vi "Enumerate Compute Nodes.vi"(8 "error in":errorcluster, 11 "request data":T3) -> (0 "error out":errorcluster, 3 "response data":T1)   [LabVIEW 2021, in "NI Discovery V1 Client.lvlib"]
uses:
  NI Discovery V1 Client.lvlib
  TypeDefs/gRPC Client Cache FGV Action.ctl
  gRPC/Generated APIs/ni/measurementlink/discovery/v1/ni.measurementlink.discovery.v1.api.lvlib
  gRPC/Generated APIs/ni/measurementlink/discovery/v1/RPC Messages/ni_measurementlink_discovery_v1_EnumerateComputeNodesRequest.ctl
  gRPC/Generated APIs/ni/measurementlink/discovery/v1/RPC Messages/ni_measurementlink_discovery_v1_ComputeNodeDescriptor.ctl
  gRPC/Generated APIs/ni/measurementlink/discovery/v1/RPC Messages/ni_measurementlink_discovery_v1_EnumerateComputeNodesResponse.ctl
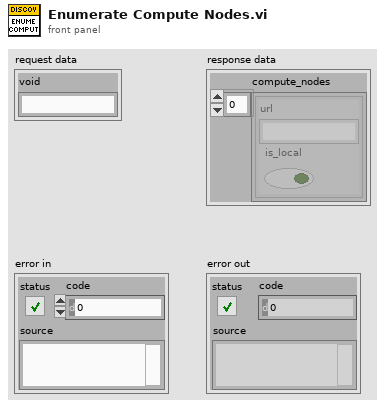
[diagram p1: front panel]
types:
  T1 = typedef "ni.measurementlink.discovery.v1.api.lvlib/ni_measurementlink_discovery_v1_EnumerateComputeNodesResponse.ctl" = cluster{"compute_nodes":T2[]}
  T2 = typedef "ni.measurementlink.discovery.v1.api.lvlib/ni_measurementlink_discovery_v1_ComputeNodeDescriptor.ctl" = cluster{"url":string, "is_local":bool}
  T3 = typedef "ni.measurementlink.discovery.v1.api.lvlib/ni_measurementlink_discovery_v1_EnumerateComputeNodesRequest.ctl" = cluster{"void":string}
  T4 = typedef "NI Discovery V1 Client.lvlib/gRPC Client Cache FGV Action.ctl" = enum16{"Get Client", "Recreate Client", "Destroy Client", "Update ClusterId"}
  T5 = typedef "grpc-lvsupport-release.lvlib/grpcId.ctl" = u64
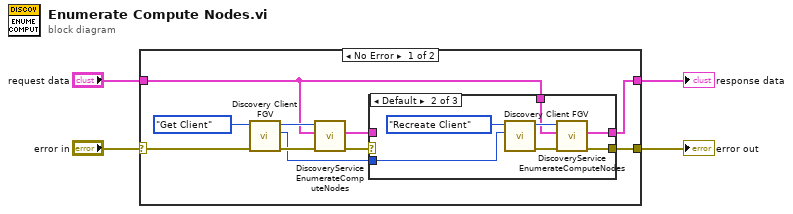
[diagram p0: block diagram]
diagram:
  n1 = case shown="No Error" "error in" {
    selector: "error in" -> [w14 w24]
    tunnel: [w9 w24] -> w3
    tunnel: [w8 _] -> w1
    tunnel: "request data" -> [w5 _]
    frame No Error {
      n2 = call "Discovery Client FGV.vi"("error in"=w14, "action"=gRPC_Client_Cache_FGV_Action."Get Client") -> ("error out"=w12:errorcluster, "unique id out"=w6:u64, "grpc client id"=w11:T5)  [unwired: 6 in, 1 out]
      n3 = call "DiscoveryService EnumerateComputeNodes.vi"("error in"=w12, "Request Data"=w5, "gRPC ID"=w11) -> ("error out"=w10:errorcluster, "Response Data"=w7:T1)  [unwired: 6 in, 1 out]
      n4 = case shown="Default" w10 {
        selector: w10 -> [w16 _ _]
        tunnel: [w16 w20 _] -> w9
        tunnel: [w15 w19 _] -> w8
        tunnel: w7 -> [w15 _ _]
        tunnel: w5 -> [_ w18 _]
        tunnel: w6 -> [_ w17 _]
        frame No Error {
        }
        frame Default {
          n5 = call "Discovery Client FGV.vi"("unique id in"=w17, "action"=gRPC_Client_Cache_FGV_Action."Recreate Client") -> ("error out"=w21:errorcluster, "grpc client id"=w22:T5)  [unwired: 6 in, 2 out]
          n6 = call "DiscoveryService EnumerateComputeNodes.vi"("error in"=w21, "Request Data"=w18, "gRPC ID"=w22) -> ("error out"=w20:errorcluster, "Response Data"=w19:T1)  [unwired: 6 in, 1 out]
        }
        frame Error {
          # "Handle UNIMPLEMENTED\noperation error by returning\nno compute nodes."
        }
      }
    }
    frame Error {
    }
  }
  "error out" <- w3
  "response data" <- w1
